vi "AnalogDemultiplexer_NI5771_HostTestvi.vi"() -> ()   [LabVIEW 2012]
uses:
  <vilib>/FPGAPlugInAG/PXIe-7962R/niLvFpga_Open_PXIe-7962R.vi
  <vilib>/rvi/interface/common/dynamic/niFpgaDynamicAddResources.vi
  <vilib>/Utility/error.llb/Error Cluster From Error Code.vi
  <vilib>/rvi/errors/niLvFpgaAdjustHostInterfaceError.vi
  <vilib>/FPGAPlugInAG/Dynamic/niLvFpga_Close_Dynamic.vi
  <vilib>/rvi/interface/nirviOpenFPGA/nirviOpenFPGA.xnode
  Scope/fpga_labview/FPGA Bitfiles/AnalogDemultiplexerV2_NI5771.lvbitx
  FPGAVIs/AnalogDemultiplexerV2_NI5771.vi
  <vilib>/rvi/interface/nirviReadWriteControl/nirviReadWriteControl.xnode
  <vilib>/rvi/interface/nirviCloseFPGA/nirviCloseFPGA.xnode
  <vilib>/rvi/interface/Simulation/niFpgaSimulationCallBeginRW.vi
  NiFpgaLv.dll
panel:
  in  "Quit":bool
  out "Configured?":bool
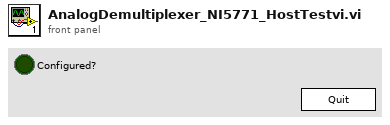
[diagram p1: front panel]
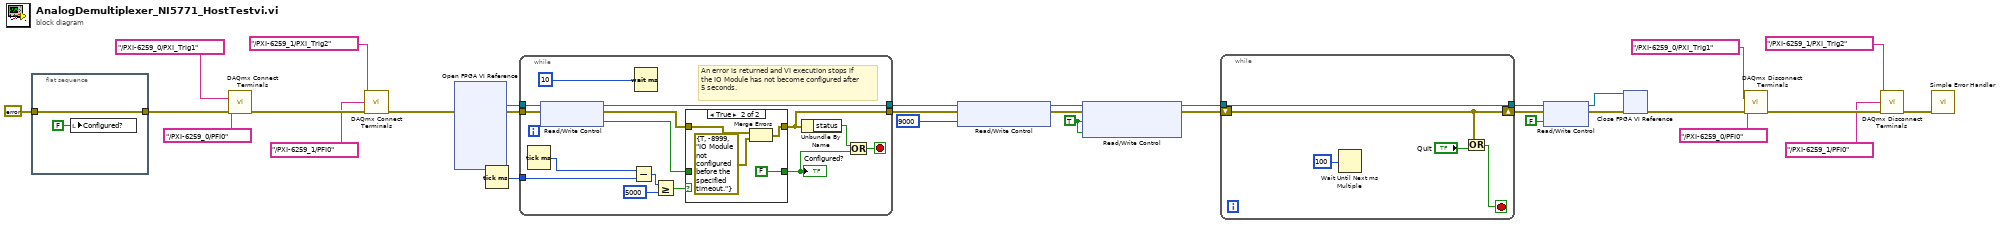
[diagram p0: block diagram]
diagram:
  w23 = TRUE ("Acquire continuously")
  n1 = flat-sequence {
    tunnel: errorcluster {"status"=FALSE, "code"=0, "source"=""} ("error in") -> [w32]
    tunnel: [w32] -> w14
    frame #0 {
      n2 = local write "Configured?"(FALSE ("Configured?")) -> ()
    }
  }
  n3 = call <vilib>:"DAQmx Connect Terminals.vi"("source terminal"=tag "/PXI-6259_0/PXI_Trig1", "destination terminal"=tag "/PXI-6259_0/PFI0", "error in"=w14) -> ("error out"=w11:errorcluster)  [unwired: 12 in]
  n4 = call <vilib>:"DAQmx Connect Terminals.vi"("source terminal"=tag "/PXI-6259_1/PXI_Trig2", "destination terminal"=tag "/PXI-6259_1/PFI0", "error in"=w11) -> ("error out"=w10:errorcluster)  [unwired: 12 in]
  n5 = xnode "Open FPGA VI Reference"("error in"=w10) -> ("FPGA VI Reference Out"=w29:refnum<k20>, "error out"=w30:errorcluster)  [unwired: 1 in]
  n6 = Tick Count (ms)() -> (millisecond timer value=w31:u32)
  n7 = while {
    tunnel: w30 -> [w41]
    tunnel: [w45] -> w28
    tunnel: [w37] -> w27
    tunnel: w29 -> [w40]
    tunnel: w31 -> [w35]
    stop <- w43 stop-if-true
    # "An error is returned and VI execution stops if the IO Module has not become configured after 5 seconds."
    n8 = Tick Count (ms)() -> (millisecond timer value=w36:u32)
    n9 = xnode "Read/Write Control"("FPGA VI Reference In"=w40, "error in"=w41) -> ("FPGA VI Reference Out"=w37:refnum<k20>, "error out"=w38:errorcluster, "Configured?"=w39:bool)
    n10 = Subtract(x=w36, y=w35) -> (x-y=w34:u32)
    n11 = Wait (ms)(milliseconds to wait=u32 10) -> ()  [unwired: 1 out]
    n12 = Greater Or Equal?(x=w34, y=u32 5000) -> (x >= y?=w46:bool)
    n13 = case shown="True" w46 {
      tunnel: [w50 FALSE ("Configured?")] -> w42
      tunnel: w39 -> [w50 _]
      tunnel: [w49 w53] -> w45
      tunnel: w38 -> [w49 w51]
      frame False {
      }
      frame True {
        n14 = Merge Errors(w51, errorcluster {"status"=TRUE, "code"=-8999, "source"="IO Module not configured before the specified timeout."} ("error in")) -> (w53:errorcluster)
      }
    }
    "Configured?" <- w42
    n15 = Unbundle By Name(w45) -> ("status"=w44:bool)
    n16 = Or(x=w44, y=w42) -> (x .or. y?=w43:bool)
  }
  n17 = xnode "Read/Write Control"("FPGA VI Reference In"=w27, "error in"=w28, "Requested pixels A1"=u16 9000 ("Samples per pixel A1")) -> ("FPGA VI Reference Out"=w24:refnum<k20>, "error out"=w25:errorcluster)
  n18 = xnode "Read/Write Control"("FPGA VI Reference In"=w24, "error in"=w25, "Acquire continuously"=w23, "Acquire"=w23) -> ("FPGA VI Reference Out"=w21:refnum<k20>, "error out"=w22:errorcluster)
  n19 = while {
    tunnel: w21 -> [w55]
    shift-right: [w59] -> w20
    shift-left: w22 -> [w59]
    tunnel: [w55] -> w19
    stop <- w58 stop-if-true
    n20 = Wait Until Next ms Multiple(millisecond multiple=u32 100) -> ()  [unwired: 1 out]
    n21 = Or(x=w59, y="Quit") -> (x .or. y?=w58:bool)
  }
  n22 = xnode "Read/Write Control"("FPGA VI Reference In"=w19, "error in"=w20, "Acquire"=FALSE) -> ("FPGA VI Reference Out"=w16:refnum<k20>, "error out"=w17:errorcluster)
  n23 = xnode "Close FPGA VI Reference"("FPGA VI Reference In"=w16, "error in"=w17) -> ("error out"=w3:errorcluster)
  n24 = call <vilib>:"DAQmx Disconnect Terminals.vi"("source terminal"=tag "/PXI-6259_0/PXI_Trig1", "destination terminal"=tag "/PXI-6259_0/PFI0", "error in"=w3) -> ("error out"=w6:errorcluster)  [unwired: 12 in]
  n25 = call <vilib>:"DAQmx Disconnect Terminals.vi"("source terminal"=tag "/PXI-6259_1/PXI_Trig2", "destination terminal"=tag "/PXI-6259_1/PFI0", "error in"=w6) -> ("error out"=w1:errorcluster)  [unwired: 12 in]
  n26 = call <vilib>:"Simple Error Handler.vi"("error in (no error)"=w1) -> ()  [unwired: 4 in, 5 out]
